vi "Stopwatch Tester.vi"() -> ()   [LabVIEW 2010]
uses:
  Stopwatch Action.ctl
panel:
  in  "Refresh":bool
  in  "Pause":bool
  in  "Start":bool
  in  "stop":bool
  out "Paused?":bool
  out "Elapsed Time":dbl
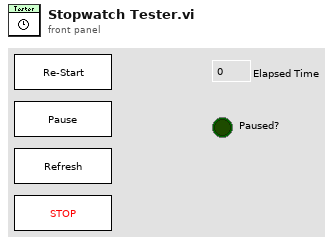
[diagram p1: front panel]
types:
  T1 = typedef "Stopwatch Action.ctl" = enum16{"Start", "Current Time", "Pause", "Reset"}
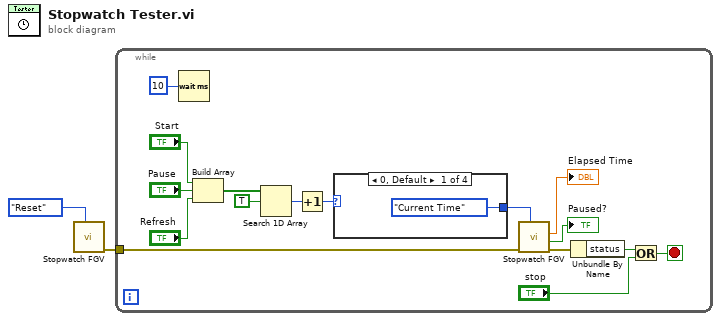
[diagram p0: block diagram]
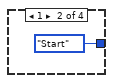
[diagram p2: hidden frame]
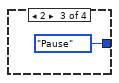
[diagram p3: hidden frame]
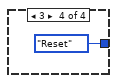
[diagram p4: hidden frame]
diagram:
  n1 = call "Stopwatch FGV.vi"("Stopwatch Action"=Stopwatch_Action."Reset") -> ("Error Out"=w2:errorcluster)  [unwired: 8 in, 2 out]
  n2 = while {
    tunnel: w2 -> [w12]
    stop <- w16 stop-if-true
    n3 = Wait (ms)(milliseconds to wait=u32 10) -> ()  [unwired: 1 out]
    n4 = Build Array("Start", "Pause", "Refresh") -> (w8:bool[])
    n5 = Search 1D Array(1D array=w8, element=TRUE) -> (index of element=w10:i32)  [unwired: 1 in]
    n6 = Increment(x=w10) -> (x+1=w11:i32)
    n7 = case shown="0, Default" w11 {
      tunnel: [Stopwatch_Action."Current Time" ("Stopwatch Action") Stopwatch_Action."Start" ("Stopwatch Action") Stopwatch_Action."Pause" ("Stopwatch Action") Stopwatch_Action."Reset" ("Stopwatch Action")] -> w4
      frame 0, Default {
      }
      frame 1 {
      }
      frame 2 {
      }
      frame 3 {
      }
    }
    n8 = call "Stopwatch FGV.vi"("Stopwatch Action"=w4, "Error In"=w12) -> ("Error Out"=w14:errorcluster, "Paused?"=→"Paused?":bool, "Elapsed Time"=→"Elapsed Time":dbl)  [unwired: 7 in]
    n9 = Unbundle By Name(w14) -> ("status"=w3:bool)
    n10 = Or(x=w3, y="stop") -> (x .or. y?=w16:bool)
  }
